vi "opencvSegmentTest.vi"() -> ()   [LabVIEW 2017]
uses:
  <vilib>/Analysis/baseanly.llb/Mean (DBL).vi
  <vilib>/Analysis/NI_AALBase.lvlib
  dll/wormUtilities/x64/Release/wormUtilities.dll
panel:
  out "Intensity Graph 3":u16[][](graph)
  out "Intensity Graph 2":i16[][](graph)
  out "Numeric":u16
  out "mean":dbl format="%0.9f"
  in  "stop":bool
  out "Intensity Graph":sgl[][](graph)
  # "TIME THE SEGMENTATION"
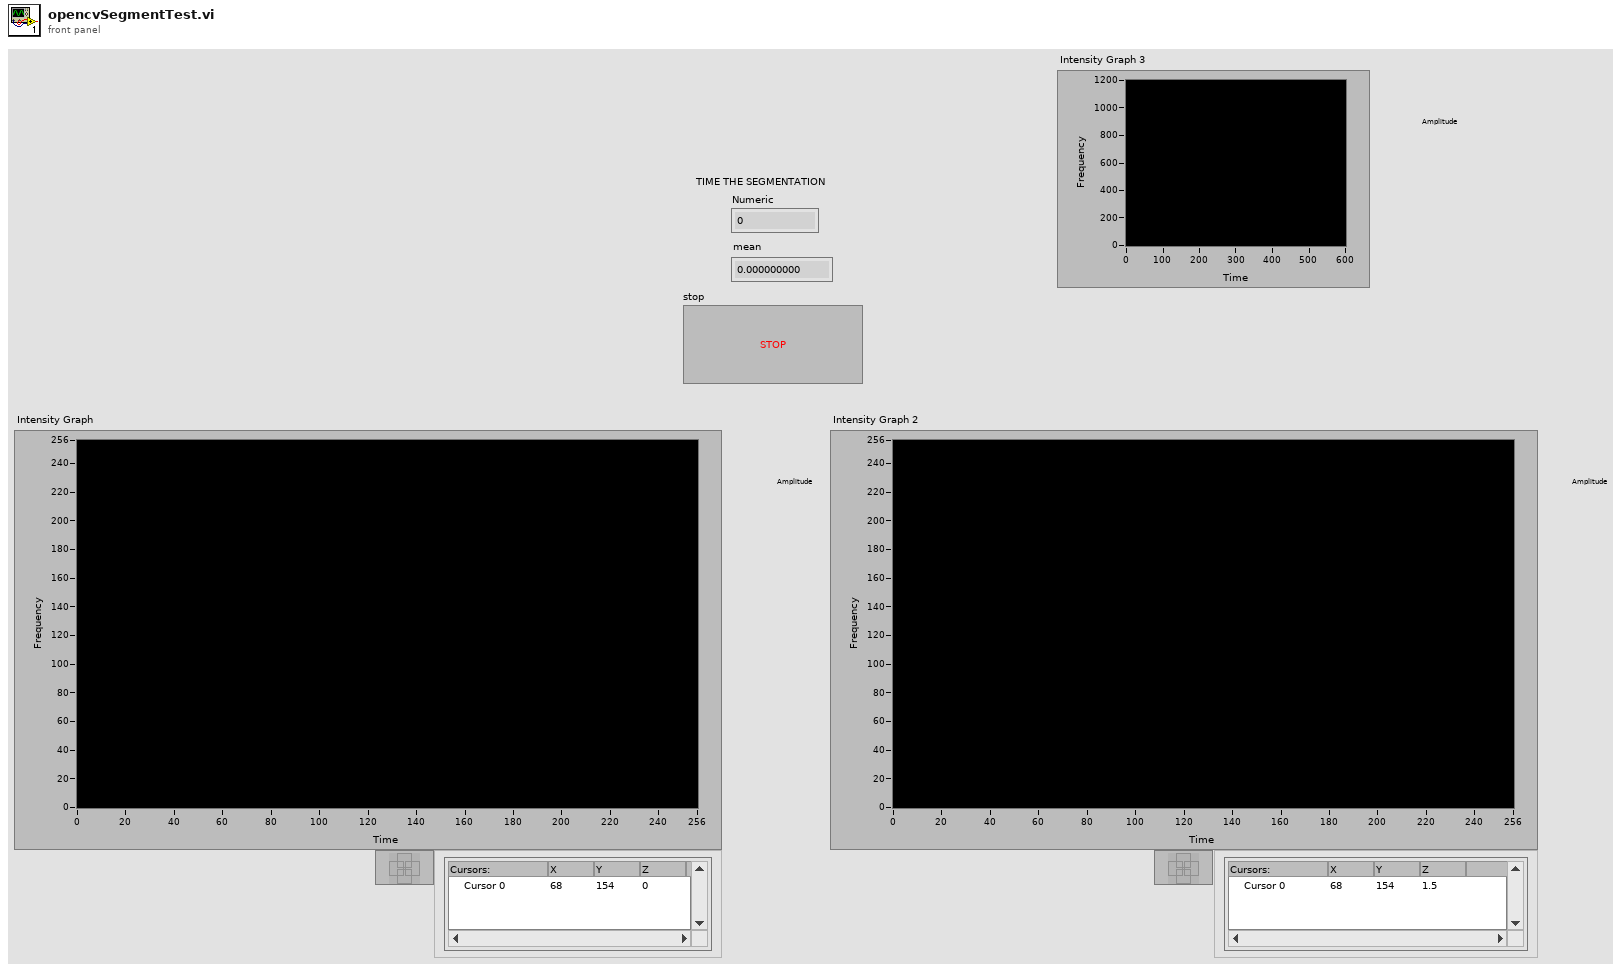
[diagram p1: front panel]
types:
  T1 = enum16{"big-endian, network order", "native, host order", "little-endian"}
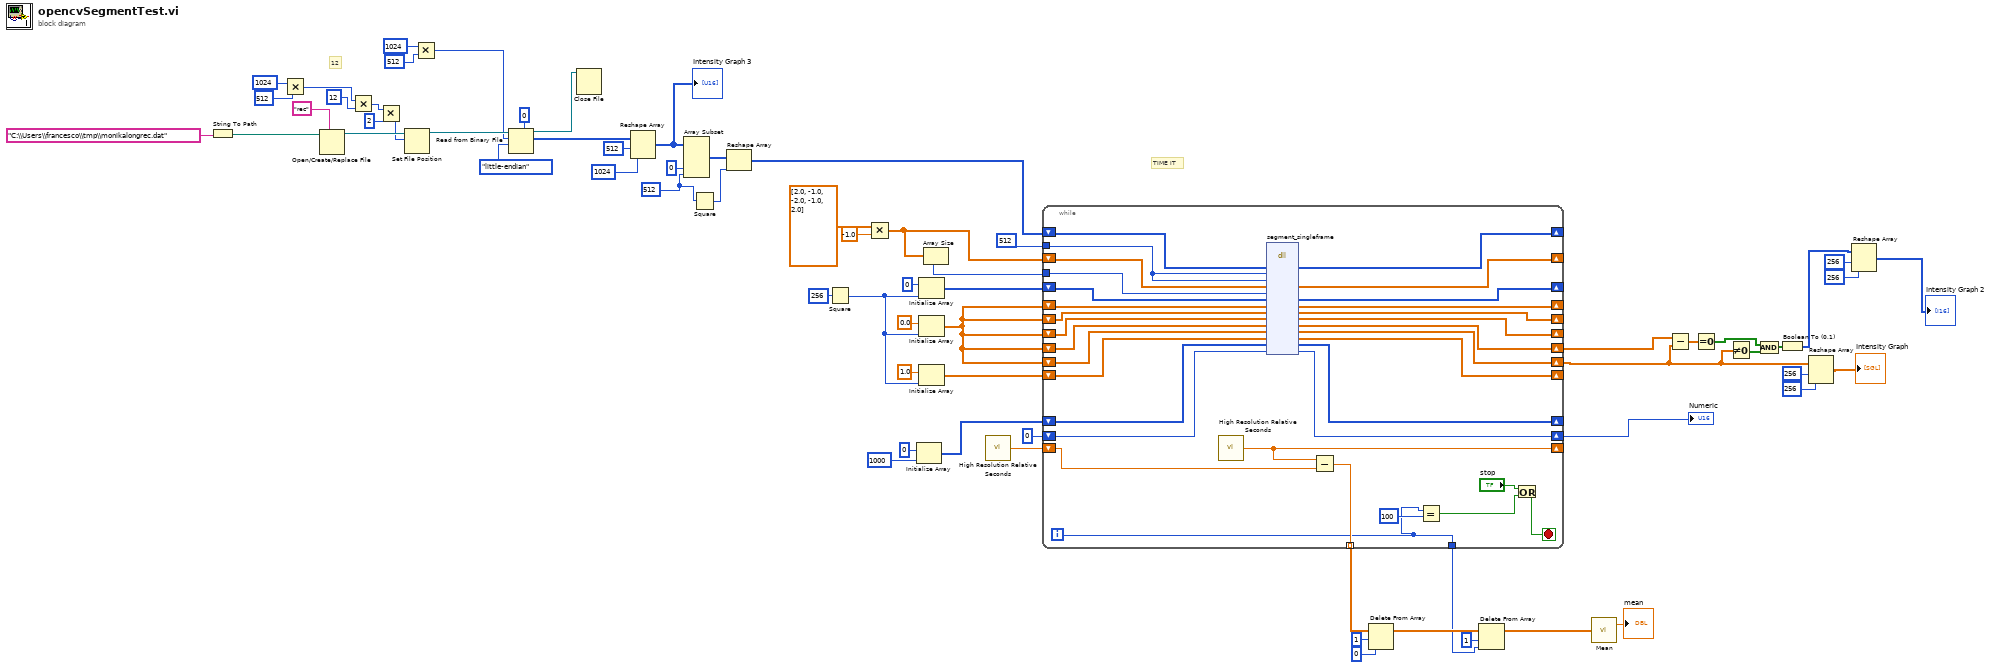
[diagram p0: block diagram]
diagram:
  w55 = 512 ("length")
  # "12"
  # "TIME IT"
  n1 = String To Path(string="C:\\Users\\francesco\\tmp\\monikalongrec.dat") -> (path=w41:path)
  n2 = Multiply(x=i64 1024, y=i64 512) -> (x*y=w59:i64)
  n3 = Open/Create/Replace File(file path (use dialog)=w41, prompt="rec") -> (refnum out=w60:refnum<file>)  [unwired: 4 in, 2 out]
  n4 = Multiply(x=w59, y=i64 12) -> (x*y=w10:i64)
  n5 = Multiply(x=w10, y=i64 2) -> (x*y=w8:i64)
  n6 = Set File Position(offset (in bytes) (0)=w8, refnum=w60) -> (refnum out=w57:refnum<file>)  [unwired: 2 in, 1 out]
  n7 = Multiply(x=1024, y=512) -> (x*y=w4:i32)
  n8 = Read from Binary File(5:u16 0, 9:T1."little-endian" ("byte order (0:big-endian, network order)"), 10:w4, 11:w57) -> (2:w61:u16[], 3:w11:refnum<file>)  [unwired: 2 in, 2 out]
  n9 = Close File(refnum=w11) -> ()  [unwired: 1 in, 2 out]
  n10 = Reshape Array(w61, 512 ("dimension size"), 1024 ("dimension size")) -> (w2:u16[][])
  "Intensity Graph 3" <- w2
  n11 = Array Subset(array=w2, index (col)=0 ("index"), length (col)=w55) -> (w53:u16[][])  [unwired: 2 in]
  n12 = Square(x=w55) -> (x^2=w54:i32)
  n13 = Reshape Array(w53, w54) -> (w40:u16[])
  n14 = Square(x=256) -> (x^2=w46:i32)
  n15 = Multiply(x=sgl[] [2.0, -1.0, -2.0, -1.0, 2.0], y=sgl -1.0) -> (x*y=w39:sgl[])
  n16 = Initialize Array(u16 0 ("element"), 1000 ("dimension size")) -> (w22:u16[])
  n17 = Initialize Array(u16 0 ("element"), w46) -> (w38:u16[])
  n18 = Initialize Array(sgl 0.0 ("element"), w46) -> (w35:sgl[])
  n19 = Initialize Array(sgl 1.0 ("element"), w46) -> (w37:sgl[])
  n20 = Array Size(array=w39) -> (size(s)=w43:i32)
  n21 = call <vilib>:"High Resolution Relative Seconds.vi"() -> ("relative seconds"=w34:dbl)
  n22 = while {
    tunnel: 512 ("sizex") -> [w93]
    shift-right: [w88] -> _
    shift-left: w40 -> [w98]
    shift-right: [w87] -> _
    shift-left: w39 -> [w97]
    shift-right: [w86] -> _
    shift-left: w38 -> [w96]
    shift-right: [w77] -> _
    shift-left: w35 -> [w95]
    shift-right: [w85] -> _
    shift-left: w35 -> [w92]
    shift-right: [w84] -> _
    shift-left: w35 -> [w91]
    shift-right: [w83] -> w18
    shift-left: w35 -> [w90]
    shift-right: [w82] -> w17
    shift-left: w35 -> [w89]
    tunnel: w43 -> [w99]
    shift-right: [w81] -> _
    shift-left: w37 -> [w94]
    shift-right: [w79] -> _
    shift-left: w34 -> [w80]
    tunnel: [w78] -> w33 mode=indexing
    tunnel: [w72] -> w27
    shift-right: [w75] -> _
    shift-left: w22 -> [w76]
    shift-right: [w68] -> w6
    shift-left: u16 0 -> [w69]
    i -> [w72]
    stop <- w70 stop-if-true
    n23 = call <vilib>:"High Resolution Relative Seconds.vi"() -> ("relative seconds"=w79:dbl)
    n24 = dll-call lib="C:/Users/francesco/dev/pump-probe/dll/wormUtilities/x64/Release/wormUtilities.dll" fn="segment_singleframe"("ImgIn"=w98, "sizex"=w93, "sizey"=w93, "arrC"=w97, "sizeC"=w99, "ArrA"=w96, "ArrB"=w95, "ArrBX"=w92, "ArrBY"=w91, "ArrBth"=w90, "ArrBdil"=w89, "ArrUno"=w94, "NeuronXY"=w76, "NeuronN"=w69) -> ("ImgIn"=w88:u16[], "arrC"=w87:sgl[], "ArrA"=w86:u16[], "ArrB"=w77:sgl[], "ArrBX"=w85:sgl[], "ArrBY"=w84:sgl[], "ArrBth"=w83:sgl[], "ArrBdil"=w82:sgl[], "ArrUno"=w81:sgl[], "NeuronXY"=w75:u16[], "NeuronN"=w68:u16)  [unwired: 7 in, 2 out]
    n25 = Subtract(x=w79, y=w80) -> (x-y=w78:dbl)
    n26 = Equal?(x=w72, y=100) -> (x = y?=w71:bool)
    n27 = Or(x="stop", y=w71) -> (x .or. y?=w70:bool)
  }
  "Numeric" <- w6
  n28 = Delete From Array(array=w33, length=1, index=0) -> (array with subset deleted=w29:dbl[])  [unwired: 1 out]
  n29 = Delete From Array(array=w29, length=1, index=w27) -> (array with subset deleted=w26:dbl[])  [unwired: 1 out]
  n30 = call-poly <vilib>:"Mean.vi"("X"=w26) -> ("mean"=→"mean":dbl)  [unwired: 1 out]
  n31 = Subtract(x=w18, y=w17) -> (x-y=w19:sgl[])
  n32 = Equal To 0?(x=w19) -> (x = 0?=w15:bool[])
  n33 = Not Equal To 0?(x=w17) -> (x != 0?=w16:bool[])
  n34 = And(x=w15, y=w16) -> (x .and. y?=w14:bool[])
  n35 = Boolean To (0,1)(Boolean=w14) -> (0, 1=w13:i16[])
  n36 = Reshape Array(w17, 256 ("dimension size"), 256 ("dimension size")) -> (→"Intensity Graph":sgl[][])
  n37 = Reshape Array(w13, 256 ("dimension size"), 256 ("dimension size")) -> (→"Intensity Graph 2":i16[][])
